vi "Update Table.vi"(8 "error in (no error)":errorcluster, 11 "DAQ970 in":refnum<class "DAQ970.lvclass">) -> (0 "error out":errorcluster, 3 "DAQ970 out":refnum<class "DAQ970.lvclass">)   [LabVIEW 2019, in "DAQ970.lvlib" / "DAQ970.lvclass"]
uses:
  Library/DAQ970.lvclass
  C:/Users/Public/Documents/Development/builds/Instruments/Instruments.lvlibp/Library/Instruments.lvclass
  Library/DAQ970.lvclass/DAQ970.ctl
  builds/Instruments/Instruments.lvlibp/Accessors/Read Measured.vi
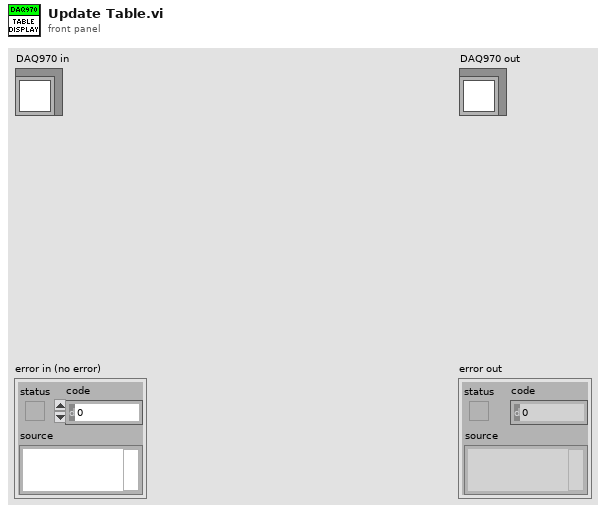
[diagram p1: front panel]
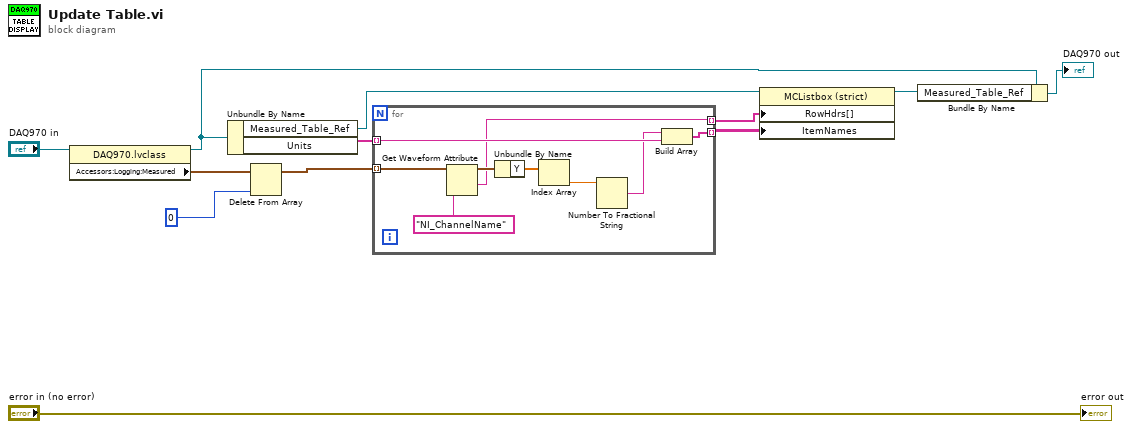
[diagram p0: block diagram]
diagram:
  n1 = property class="DAQ970.lvclass"(reference="DAQ970 in") -> (reference out=w9:refnum<class "DAQ970.lvclass">, "Accessors:Logging:Measured"=w11:waveform(dbl)[])  [unwired: 1 in, 1 out]
  n2 = Unbundle By Name(w9) -> ("Measured_Table_Ref"=w3:refnum<vi>, "Units"=w7:string[])
  n3 = Delete From Array(array=w11, index=0) -> (array with subset deleted=w8:waveform(dbl)[])  [unwired: 1 in, 1 out]
  n4 = for {
    tunnel: w8 -> [w21] mode=indexing
    tunnel: w7 -> [w16] mode=indexing
    tunnel: [w14] -> w1 mode=indexing
    tunnel: [w13] -> w2 mode=indexing
    w20 = "NI_ChannelName" ("name")
    n5 = Get Waveform Attribute(5:w20, 6:w20, 7:w21) -> (1:w13:string, 3:w19:waveform(dbl))  [unwired: 1 in, 2 out]
    n6 = Unbundle By Name(w19) -> ("Y"=w18:dbl[])
    n7 = Index Array(array=w18) -> (element=w17:dbl)  [unwired: 1 in]
    n8 = Number To Fractional String(number=w17) -> (F-format string=w15:string)  [unwired: 3 in]
    n9 = Build Array(w15, w16) -> (w14:string[])
  }
  n10 = property class="MCListbox (strict)"(reference=w3, "RowHdrs[]"=w2, "ItemNames"=w1) -> (reference out=w4:refnum<vi>)  [unwired: 1 in, 1 out]
  n11 = Bundle By Name(cluster=w9, "Measured_Table_Ref"=w4) -> (→"DAQ970 out":refnum<class "DAQ970.lvclass">)
  "error out" <- "error in (no error)"
